vi "hostCommander_old1.vi"() -> ()   [LabVIEW 2014]
uses:
  <vilib>/platform/TimedLoop/XDataNode/XDataNode.xnode
  <vilib>/Platform/TimedLoop/XDataNode/nitl_modes.ctl
  <vilib>/Platform/TimedLoop/XDataNode/XDNodeRunTimeDep.lvlib
  <vilib>/Platform/TimedLoop/XDataNode/wakeup.ctl
  <vilib>/Platform/TimedLoop/XDataNode/timing_clust.ctl
  UDP_Para_def.ctl
panel:
  out "DigitalWaveformGraph":digitalwaveform(graph)={"t0"=timestamp(10 s since 1904-01-01), "dt"=0.002, "Y"={"transitions"=[], "data"=array5000x7[35000 elements]}, "error"={"status"=FALSE, "code"=37421928, "source"=""}} caption="Digital Waveform Graph"
  out "Current state":T1(ring)=enum."Before VS"
  out "Trial #":u32=1
  out "Sec":dbl=42.04900000000001
  out "Min":dbl=1.0
  out "Busy":bool
  out "Trial # (host)":u32=1
  out "stateLatched":bool
  in  "statusDispLength (S)":sgl=10.0
  in  "stateParaCluster":T2={"rtFIFOarraySize"=50, "rtFIFOsize"=50, "rtFIFOname1"="", "rtFIFOtimeout"=0.0, "rtFIFOname2"="", "shockOn_uS"=0, "timeout_uS"=0, "waterOn_uS"=0, "rewardTimeWindow_uS "=0, "stateMachineCycle_uS"=500}
  in  "channelParaCluster":T3={"vsFilterPeriod"=500, "lickThreshold"=0.0, "vsThreshold"=0.0, "audioThreshold_V"=0.009002685546875, "audioFilterPeriod_uS"=50000, "audioOffState_V"=-0.0035}
  out "error out":errorcluster
  in  "Stop state":bool
  in  "ABORT":bool
  in  "Remote port":u16=9090
  in  "Remote IP_Main":string="192.168.137.1"
  in  "Local port":u16=9091
  in  "Local IP_RT":string="192.168.137.2"
  out "Actual":i64=11
  in  "File name":string="91014_14-2_2"
  in  "Save file to":string="C:\\ni-rt\\LabVIEW Data\\"
  in  "Save data":bool
  out "Rewards #":i32
  out "RT FIFO (DISP)":u32(slide) scale=0.0..50.0
  out "RT FIFO (Log)":u32(slide) scale=0.0..50.0
  # "Elapsed time"
  # "Sec"
  # "Min"
  # "Controls"
  # "Network"
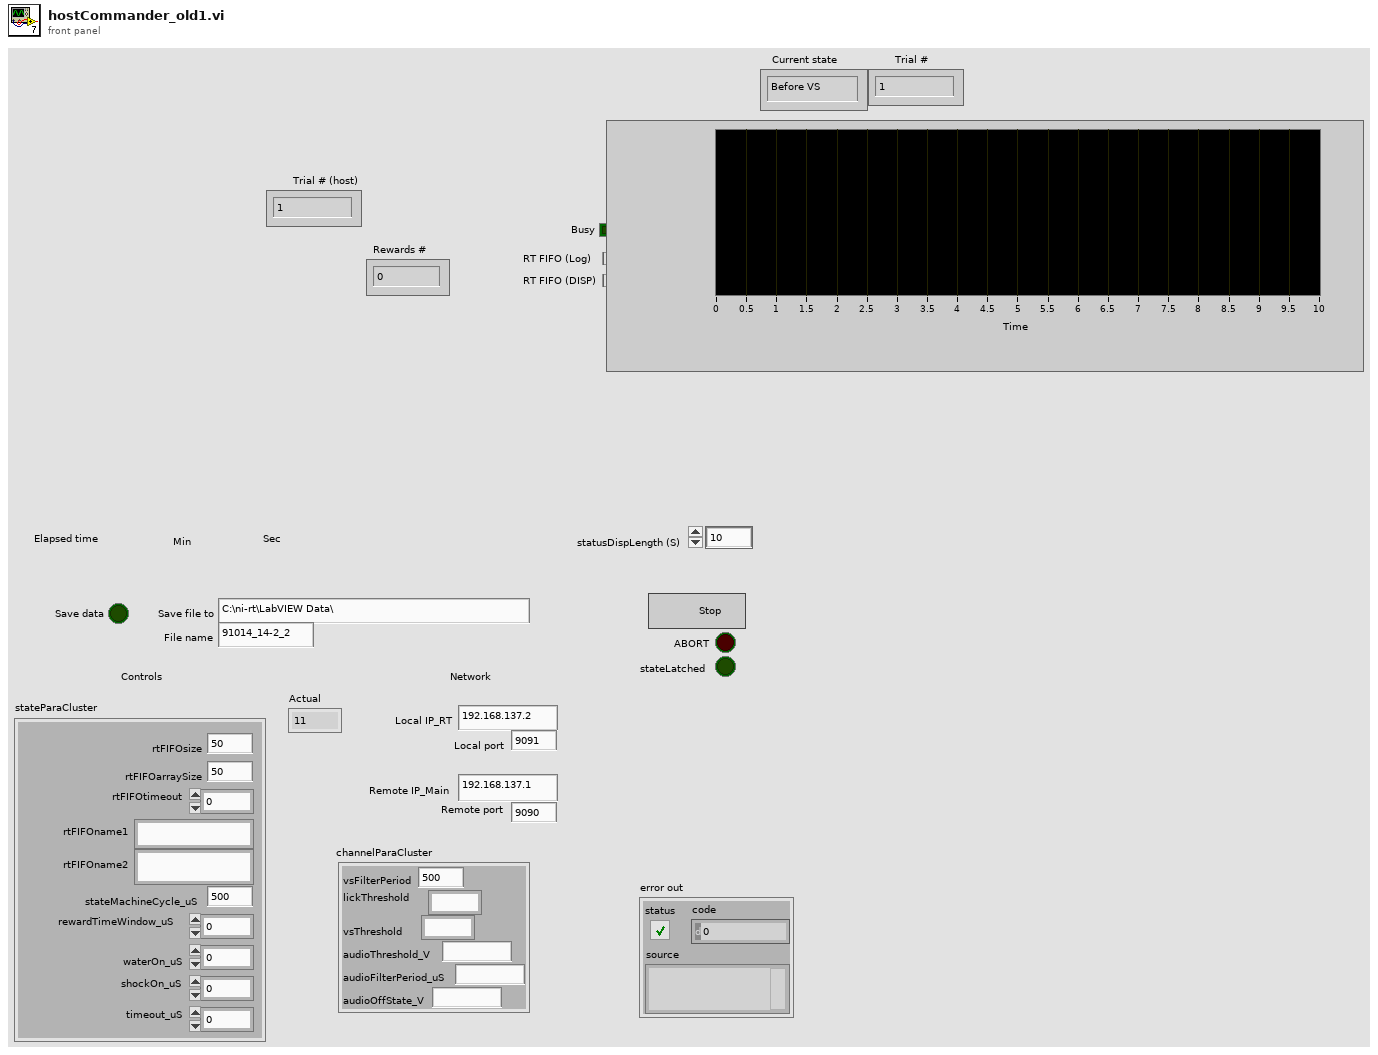
[diagram p1: front panel]
types:
  T1 = enum16{"Idle", "Before VS", "VS", "After VS", "Cycle End", "Reward", "Reward Refractory", "Punish", "Punish Refractory", "Exit", "Timeout", "Lick reward"}
  T2 = cluster{"rtFIFOarraySize":u32, "rtFIFOsize":u32, "rtFIFOname1":string, "rtFIFOtimeout":dbl, "rtFIFOname2":string, "shockOn_uS":i32, "timeout_uS":i32, "waterOn_uS":i32, "rewardTimeWindow_uS ":i32, "stateMachineCycle_uS":i64}
  T3 = cluster{"vsFilterPeriod":i64, "lickThreshold":fxp<+/-,16,5>, "vsThreshold":fxp<+/-,16,5>, "audioThreshold_V":fxp<+/-,32,16>, "audioFilterPeriod_uS":i32, "audioOffState_V":dbl}
  T4 = typedef "XDNodeRunTimeDep.lvlib/timing_clust.ctl" = cluster{"Expected End [f-1]":u64, "Actual End [f-1]":u64, "Finished Late? [f-1]":bool, "Expected End [i-1]":u64, "Actual End [i-1]":u64, "Finished Late? [i-1]":bool, "Expected Start [i]":u64, "Actual Start [i]":u64, "Expected Start [f]":u64, "Actual Start [f]":u64, "Source Name":string, "Structure Name":string, "Period":i64, "Deadline":i64, "Offset":i64, "Start":i64, "Priority":i32, "Timeout":i32, "Mode":T5, "Wakeup Reason":T6, "Error":errorcluster, "Source Type":string, "Secondary Source Type":string, "Global End Time":u64, "Global Start Time":u64, "Frame Duration":u64, "Iteration Duration":u64, "Assigned CPU":i32, "I/O Scan Engine Mode":u32}
  T5 = typedef "XDNodeRunTimeDep.lvlib/nitl_modes.ctl" = enum32{"No Change", "Process missed periods, maintain original phase", "Discard missed periods, maintain original phase", "Process missed periods, ignore original phase", "Discard missed periods, ignore original phase"}
  T6 = typedef "XDNodeRunTimeDep.lvlib/wakeup.ctl" = enum32{"Normal", "Aborted", "Asynchronous wakeup", "Timing source error", "Timed loop error", "Timeout"}
  T7 = typedef "UDP_Para_def.ctl" = enum16{"no", "start", "stop", "dly", "rwp", "rwf", "wdr", "shd", "tod", "lkr", "tlr", "alp", "msh", "mwl", "mwr", "lth", "vth", "ath", "aof", "afp", "vfp"}
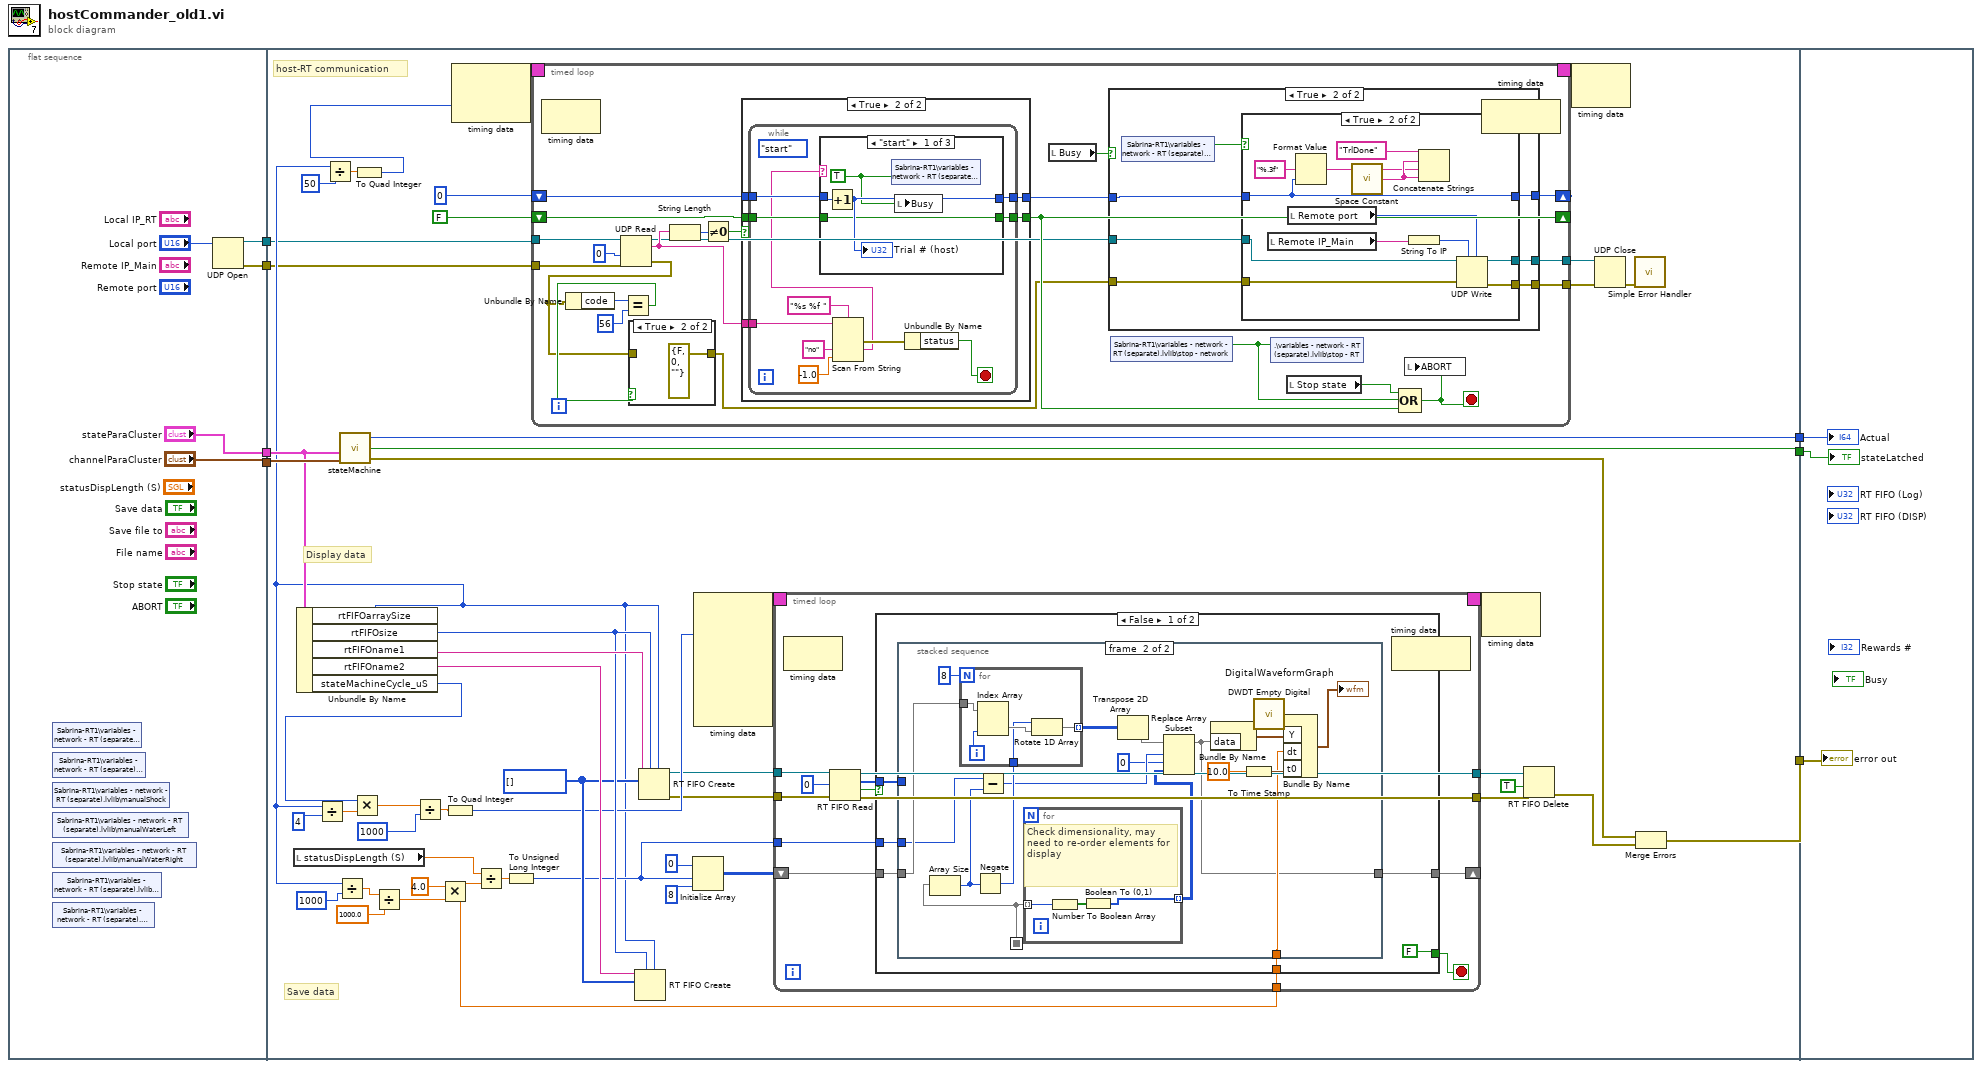
[diagram p0: block diagram]
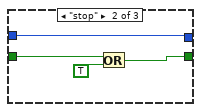
[diagram p5: hidden frame]
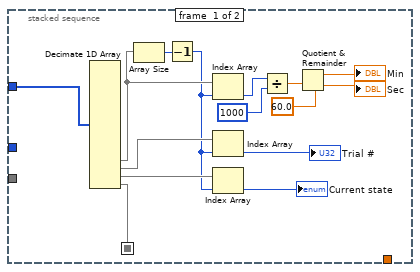
[diagram p8: hidden frame]
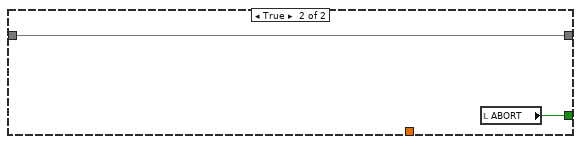
[diagram p9: hidden frame]
diagram:
  n1 = flat-sequence {
    tunnel: ["stateParaCluster"] -> w7
    tunnel: ["channelParaCluster"] -> w6
    tunnel: [w9] -> w2
    tunnel: [w8] -> w1
    tunnel: w7 -> [w31]
    tunnel: w6 -> [w32]
    tunnel: [w30] -> w5
    tunnel: [w29] -> w4
    tunnel: [w27] -> w3
    tunnel: w2 -> [w19]
    tunnel: w1 -> [w18]
    tunnel: w5 -> [w216]
    tunnel: w4 -> [w215]
    tunnel: w3 -> [w214]
    frame #0 {
      n2 = shared-variable "Sabrina-RT1\\variables - network - RT (separate).lvlib\\trailStart"() -> ()  [unwired: 1 in, 2 out]
      n3 = shared-variable "Sabrina-RT1\\variables - network - RT (separate).lvlib\\trailDone"() -> ()  [unwired: 1 in, 2 out]
      n4 = shared-variable "Sabrina-RT1\\variables - network - RT (separate).lvlib\\manualShock"() -> ()  [unwired: 1 in, 2 out]
      n5 = shared-variable "Sabrina-RT1\\variables - network - RT (separate).lvlib\\manualWaterLeft"() -> ()  [unwired: 1 in, 2 out]
      n6 = shared-variable "Sabrina-RT1\\variables - network - RT (separate).lvlib\\manualWaterRight"() -> ()  [unwired: 1 in, 2 out]
      n7 = shared-variable "Sabrina-RT1\\variables - network - RT (separate).lvlib\\allowPunish"() -> ()  [unwired: 1 in, 2 out]
      n8 = shared-variable "Sabrina-RT1\\variables - network - RT (separate).lvlib\\lickReward"() -> ()  [unwired: 1 in, 2 out]
      n9 = UDP Open(11:"Local port") -> (port=w9:refnum<k16>, 0:w8:errorcluster)  [unwired: 4 in, 1 out]
    }
    frame #1 {
      w59 = u32[] []
      # "host-RT communication"
      # "Save data"
      # "Display data"
      n10 = local read "statusDispLength (S)"() -> (w38:sgl)
      n11 = call "stateMachine.vi"("chanellParaCluster"=w32) -> ("error out"=w28:errorcluster, "stateLatched"=w29:bool, "actualCycle_uS"=w30:i64, "stateParaCluster"=w31:T2)  [unwired: 2 in]
      n12 = Unbundle By Name(w31) -> ("rtFIFOarraySize"=w23:u32, "rtFIFOsize"=w61:u32, "rtFIFOname1"=w62:string, "rtFIFOname2"=w60:string, "stateMachineCycle_uS"=w55:i64)
      n13 = Divide(x=w23, y=u32 4) -> (x/y=w54:dbl)
      n14 = Divide(x=w23, y=i64 50) -> (x/y=w21:dbl)
      n15 = Divide(x=w23, y=u32 1000) -> (x/y=w46:dbl)
      n16 = Multiply(x=w55, y=w54) -> (x*y=w53:dbl)
      n17 = To Quad Integer(1:w21) -> (0:w20:i64)
      n18 = Divide(x=w46, y=1000.0) -> (x/y=w44:dbl)
      n19 = Divide(x=w53, y=u32 1000) -> (x/y=w51:dbl)
      n20 = Multiply(x=4.0, y=w44) -> (x*y=w37:dbl)
      n21 = To Quad Integer(1:w51) -> (0:w50:i64)
      n22 = node-c288(w20) -> (w25:T4)  [unwired: 1 in]
      n23 = Divide(x=w38, y=w37) -> (x/y=w42:dbl)
      n24 = To Unsigned Long Integer(number=w42) -> (unsigned 32bit integer=w36:u32)
      n25 = timed-loop {
        timing: w25 -> [_]
        timing-out: [_] -> w24
        tunnel: w19 -> [w81]
        tunnel: w18 -> [w80]
        shift-right: [w74] -> _
        shift-left: 0 ("timeout ms (25000)") -> [w76]
        shift-right: [w70] -> _
        shift-left: FALSE -> [w73]
        tunnel: [w65] -> w15
        tunnel: [w64] -> w14
        stop <- w72 stop-if-true
        n26 = node-c288() -> ()  [unwired: 1 in, 1 out]
        n27 = UDP Read(connection ID=w81, timeout ms (25000)=0, 8:w80) -> (data out=w77:string, error out=w63:errorcluster, 3:w68:refnum<k16>)  [unwired: 1 in, 2 out]
        n28 = Unbundle By Name(w63) -> ("code"=w83:i32)
        n29 = Equal?(x=w83, y=56) -> (x = y?=w85:bool)
        n30 = case shown="True" w85 {
          tunnel: w63 -> [w139 _]
          tunnel: [w139 errorcluster {"status"=FALSE, "code"=0, "source"=""} ("error out")] -> w69
          frame False {
          }
          frame True {
          }
        }
        n31 = String Length(string=w77) -> (length=w79:i32)
        n32 = Not Equal To 0?(x=w79) -> (x != 0?=w78:bool)
        n33 = case shown="True" w78 {
          tunnel: w77 -> [_ w117]
          tunnel: w76 -> [w112 w116]
          tunnel: [w112 w115] -> w75
          tunnel: w73 -> [w111 w114]
          tunnel: [w111 w113] -> w70
          frame False {
          }
          frame True {
            n34 = while {
              tunnel: w117 -> [w128]
              tunnel: w116 -> [w122]
              tunnel: [w121] -> w115
              tunnel: w114 -> [w120]
              tunnel: [w119] -> w113
              stop <- w123 stop-if-true
              (unwired) UDP_Para_def."start"
              n35 = Scan From String(format string="%s %f ", input string=w128, default 1="no" ("default value 1"), default 2=-1.0 ("default value 2")) -> (error out=w124:errorcluster, output 1=w118:string)  [unwired: 3 in, 2 out]
              n36 = case shown="\"start\"" w118 {
                tunnel: [w131 w136 w138] -> w121
                tunnel: w122 -> [w132 w136 w138]
                tunnel: [w130 w133 w137] -> w119
                tunnel: w120 -> [w130 w134 w137]
                frame "start" {
                  w129 = TRUE
                  n37 = Increment(x=w132) -> (x+1=w131:i32)
                  "Trial # (host)" <- w131
                  n38 = shared-variable "Sabrina-RT1\\variables - network - RT (separate).lvlib\\trailStart"(w129) -> ()  [unwired: 1 in, 1 out]
                  n39 = local write "Busy"(w129) -> ()
                }
                frame "stop" {
                  n40 = Or(x=w134, y=TRUE) -> (x .or. y?=w133:bool)
                }
                frame "no", Default {
                }
              }
              n41 = Unbundle By Name(w124) -> ("status"=w123:bool)
            }
          }
        }
        n42 = local read "Busy"() -> (w71:bool)
        n43 = case shown="True" w71 {
          tunnel: w75 -> [w88 w95]
          tunnel: [w88 w94] -> w74
          tunnel: w69 -> [w86 w93]
          tunnel: w68 -> [w87 w92]
          tunnel: [w87 w90] -> w65
          tunnel: [w86 w89] -> w64
          frame False {
          }
          frame True {
            n44 = shared-variable "Sabrina-RT1\\variables - network - RT (separate).lvlib\\trailDone"() -> (w91:bool)  [unwired: 1 in, 1 out]
            n45 = case shown="True" w91 {
              tunnel: w95 -> [w98 w103]
              tunnel: [w98 w103] -> w94
              tunnel: w93 -> [w96 w102]
              tunnel: w92 -> [w97 w101]
              tunnel: [w97 w100] -> w90
              tunnel: [w96 w99] -> w89
              frame False {
              }
              frame True {
                n46 = local read "Remote IP_Main"() -> (w106:string)
                n47 = local read "Remote port"() -> (w105:u16)
                n48 = Format Value(format string="%.3f", value (0)=w103) -> (output string=w107:string)  [unwired: 1 in]
                n49 = call <vilib>:"Space Constant.vi"() -> ("String"=w109:string)
                n50 = String To IP(1:w106) -> (0:w104:u32)
                n51 = Concatenate Strings("TrlDone" ("data in"), w109, w107, w109) -> ()  [unwired: 1 out]
                n52 = UDP Write(address=w104, port or service name=w105, connection ID=w101, 8:w102) -> (error out=w99:errorcluster, 3:w100:refnum<k16>)  [unwired: 2 in]
              }
            }
          }
        }
        n53 = shared-variable "Sabrina-RT1\\variables - network - RT (separate).lvlib\\stop - network"() -> (w67:bool)  [unwired: 1 in, 1 out]
        n54 = shared-variable ".\\variables - network - RT (separate).lvlib\\stop - RT"(w67) -> ()  [unwired: 1 in, 1 out]
        n55 = local read "Stop state"() -> (w66:bool)
        n56 = Compound Arithmetic op=OR(w66, w67, w70) -> (w72:bool)
        n57 = local write "ABORT"(w72) -> ()
        n58 = node-c288() -> ()  [unwired: 1 in, 1 out]
      }
      n59 = RT FIFO Create(0:w60, 1:w59, 4:w61, 6:w23) -> ()  [unwired: 4 in, 3 out]
      n60 = RT FIFO Create(0:w62, 1:w59, 4:w61, 6:w23) -> (8:w49:refnum<k33>, 11:w48:errorcluster)  [unwired: 4 in, 1 out]
      n61 = Initialize Array(u8 0 ("element"), w36, 8 ("dimension size")) -> (w39:u8[][])
      n62 = node-c288(w50) -> (w58:T4)  [unwired: 6 in]
      n63 = timed-loop {
        timing: w58 -> [_]
        timing-out: [_] -> w57
        tunnel: w49 -> [w158]
        tunnel: w48 -> [w157]
        tunnel: w37 -> [w152]
        tunnel: w36 -> [w151]
        shift-right: [w150] -> _
        shift-left: w39 -> [w153]
        tunnel: [w149] -> w35
        tunnel: [w148] -> w34
        stop <- w147 stop-if-true
        n64 = node-c288() -> ()  [unwired: 1 in, 1 out]
        n65 = RT FIFO Read(0:w158, 2:0, 3:w157) -> (8:w149:refnum<k33>, 9:w154:u32[], 10:w155:bool, 11:w148:errorcluster)  [unwired: 1 in, 1 out]
        n66 = case shown="False" w155 {
          tunnel: w154 -> [w159 _]
          tunnel: w153 -> [w162 w207]
          tunnel: w152 -> [w163 _]
          tunnel: w151 -> [w161 _]
          tunnel: [w160 w207] -> w150
          tunnel: [FALSE w206] -> w147
          frame False {
            n67 = stacked-sequence {
              seq-local: [w165 _] -> [_ w180]
              tunnel: w159 -> [w179 _]
              tunnel: w162 -> [_ w194]
              tunnel: w163 -> [_ w183]
              tunnel: w161 -> [_ w182]
              tunnel: [_ w181] -> w160
              frame #0 {
                n68 = Decimate 1D Array(w179) -> (w171:u32[], w173:u32[], w174:u32[], w165:u32[])  [unwired: 12 out]
                n69 = Array Size(array=w171) -> (size(s)=w170:i32)
                n70 = Decrement(x=w170) -> (x-1=w169:i32)
                n71 = Index Array(array=w171, index=w169) -> (element=w178:u32)
                n72 = Index Array(array=w173, index=w169) -> (element=→"Trial #":u32)
                n73 = Index Array(array=w174, index=w169) -> (element=→"Current state":u32)
                n74 = Divide(x=w178, y=u32 1000) -> (x/y=w176:dbl)
                n75 = Quotient & Remainder(x=w176, y=60.0) -> (x-y*floor(x/y)=→"Min":dbl, floor(x/y)=→"Sec":dbl)
              }
              frame #1 {
                n76 = Array Size(array=w180) -> (size(s)=w197:i32)
                n77 = Negate(x=w197) -> (-x=w193:i32)
                n78 = for {
                  N: 8 -> [_]
                  tunnel: w194 -> [w202]
                  tunnel: w193 -> [w199]
                  tunnel: [w198] -> w195 mode=indexing
                  i -> [w201]
                  n79 = Index Array(array=w202, index (col)=w201) -> (element=w200:u8[])  [unwired: 1 in]
                  n80 = Rotate 1D Array(1:w200, 2:w199) -> (0:w198:u8[])
                }
                n81 = Subtract(x=w182, y=w197) -> (x-y=w187:u32)
                n82 = for {
                  tunnel: w180 -> [w203] mode=indexing
                  tunnel: [w205] -> w185 mode=indexing
                  # "Check dimensionality, may need to re-order elements for display"
                  n83 = Number To Boolean Array(number=w203) -> (Boolean array=w204:bool[])
                  n84 = Boolean To (0,1)(Boolean=w204) -> (0, 1=w205:i16[])
                }
                n85 = Transpose 2D Array(2D array=w195) -> (transposed array=w188:u8[][])
                n86 = Replace Array Subset(array=w188, new element=w185, index (row)=w187, index (col)=0 ("disabled index (col)")) -> (w181:u8[][])
                n87 = Bundle By Name("data"=w181) -> (w192:digitaldata)  [unwired: 1 in]
                n88 = To Time Stamp(1:10.0 ("number")) -> (0:w190:timestamp)
                n89 = call <vilib>:"DWDT Empty Digital.vi"() -> ("digital waveform out"=w191:digitalwaveform)  [unwired: 5 in]
                n90 = Bundle By Name(cluster=w191, "Y"=w192, "dt"=w183, "t0"=w190) -> (→"DigitalWaveformGraph":digitalwaveform)
              }
            }
          }
          frame True {
            n91 = local read "ABORT"() -> (w206:bool)
          }
        }
        n92 = node-c288() -> ()  [unwired: 1 in, 1 out]
      }
      n93 = node-c288(w57) -> ()  [unwired: 1 out]
      n94 = RT FIFO Delete(0:w35, 2:TRUE ("force destroy? (F)"), 3:w34) -> (11:w26:errorcluster)
      n95 = node-c288(w24) -> ()  [unwired: 1 out]
      n96 = UDP Close(connection ID=w15, 8:w14) -> (error out=w13:errorcluster)  [unwired: 1 out]
      n97 = call <vilib>:"Simple Error Handler.vi"("error in (no error)"=w13) -> ()  [unwired: 4 in, 5 out]
      n98 = Merge Errors(w28, w26) -> (w27:errorcluster)
    }
    frame #2 {
      "error out" <- w214
      "Actual" <- w216
      "stateLatched" <- w215
    }
  }
